vi "modify ROI without transform.vi"(8 "error in (no error)":errorcluster caption="错误输入（无错误）", 9 "new x y":cluster{"X":sgl, "Y":sgl}, 10 "ROI size":i32) -> (0 "error out":errorcluster caption="错误输出", 2 "ROI Descriptor out":T1 {"Contours"."Type" items=["No Selection", "Point", "Line", "Rectangle", "Oval", "Polygon", "Freehand Region", "Annulus", "Unused2", "Unused3", "Broken Line", "Freehand Line", "Rotated Rectangle"]})   [LabVIEW 2017]
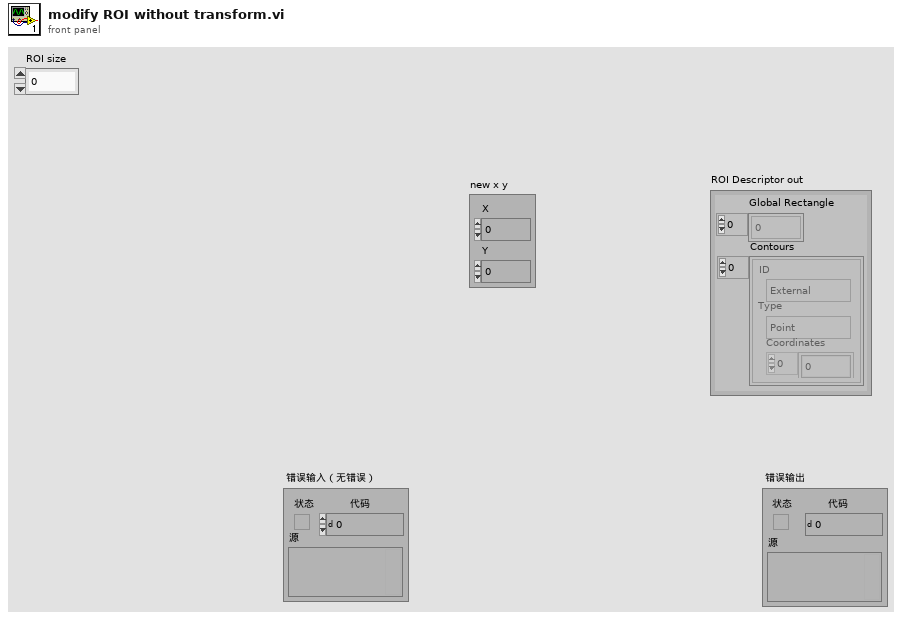
[diagram p1: front panel]
types:
  T1 = typedef "ROI Descriptor" = cluster{"Global Rectangle":i32[], "Contours":cluster{"ID":enum32{"External", "Internal"}, "Type":u32, "Coordinates":i32[]}[]}
  T2 = typedef "IMAQ Rectangle" = cluster{"Left":i32, "Top":i32, "Right":i32, "Bottom":i32, "Rotation":dbl}
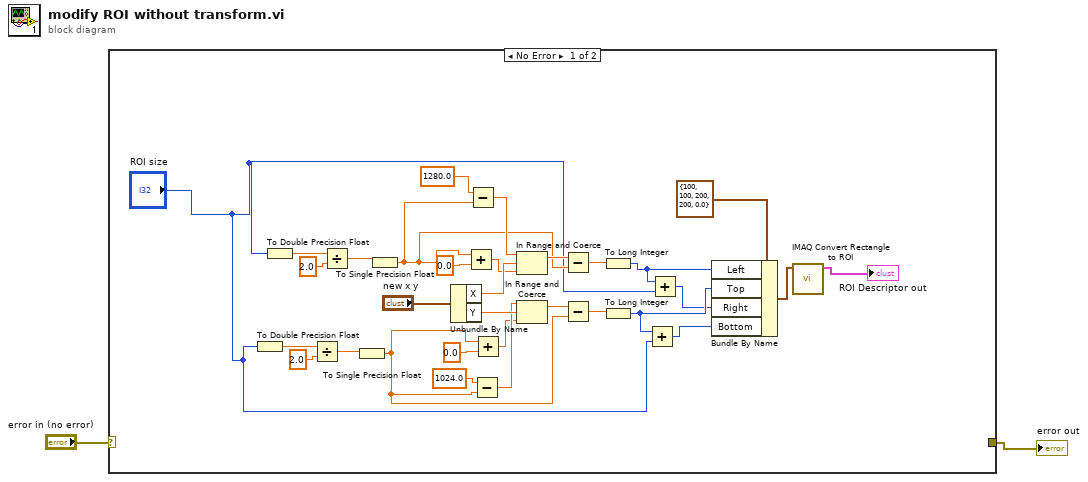
[diagram p0: block diagram]
diagram:
  n1 = case shown="No Error" "error in (no error)" {
    selector: "error in (no error)" -> [_ w34]
    tunnel: [_ w34] -> w1
    frame No Error {
      n2 = To Double Precision Float(number="ROI size") -> (double precision float=w19:dbl)
      n3 = To Double Precision Float(number="ROI size") -> (double precision float=w30:dbl)
      n4 = Divide(x=w19, y=2.0) -> (x/y=w18:dbl)
      n5 = Divide(x=w30, y=2.0) -> (x/y=w31:dbl)
      n6 = To Single Precision Float(number=w18) -> (single precision float=w13:sgl)
      n7 = To Single Precision Float(number=w31) -> (single precision float=w14:sgl)
      n8 = Unbundle By Name("new x y") -> ("X"=w29:sgl, "Y"=w27:sgl)
      n9 = Add(x=w14, y=sgl 0.0 ("下限")) -> (x+y=w15:sgl)
      n10 = Subtract(x=sgl 1280.0 ("上限"), y=w14) -> (x-y=w24:sgl)
      n11 = Subtract(x=sgl 1024.0 ("上限"), y=w13) -> (x-y=w22:sgl)
      n12 = Add(x=w13, y=sgl 0.0 ("下限")) -> (x+y=w20:sgl)
      n13 = In Range and Coerce(upper limit=w24, x=w29, lower limit=w15) -> (coerced(x)=w28:sgl)  [unwired: 1 out]
      n14 = In Range and Coerce(upper limit=w22, x=w27, lower limit=w20) -> (coerced(x)=w26:sgl)  [unwired: 1 out]
      n15 = Subtract(x=w28, y=w14) -> (x-y=w9:sgl)
      n16 = Subtract(x=w26, y=w13) -> (x-y=w8:sgl)
      n17 = To Long Integer(number=w9) -> (32bit integer=w5:i32)
      n18 = To Long Integer(number=w8) -> (32bit integer=w7:i32)
      n19 = Add(x=w7, y="ROI size") -> (x+y=w6:i32)
      n20 = Add(x=w5, y="ROI size") -> (x+y=w4:i32)
      n21 = Bundle By Name(cluster=T2 {"Left"=100, "Top"=100, "Right"=200, "Bottom"=200, "Rotation"=0.0} ("ROI size"), "Left"=w5, "Top"=w7, "Right"=w4, "Bottom"=w6) -> (w10:T2)
      n22 = call "IMAQ Convert Rectangle to ROI"("Rectangle"=w10) -> ("ROI Descriptor"=→"ROI Descriptor out":T1)  [unwired: 8 in, 1 out]
    }
    frame Error {
    }
  }
  "error out" <- w1
